vi "Get All Dispatcher Queues.vi"(0 "receiver host (\"\")":string, 5 "receiver port (0)":u16, 11 "error in":errorcluster) -> (4 "response message":T1, 6 "string response":string, 8 "queue names":string[](array[string]), 15 "error out":errorcluster)   [LabVIEW 2013, in "AMC.lvlib"]
doc: "Requests a list of all the queue names in the application instance specified by \"receiver host\" and \"receiver port\".\n\nIf \"receiver port\" is undefined, this VI will attempt to use the default UDP port."
uses:
  AMC.lvlib
  Message.ctl
  <vilib>/NI/Tools/Keyed Array/KeyedArray.ctl
  <vilib>/NI/Tools/Keyed Array/Map String.vi
  <vilib>/NI/Tools/String/Get Case Matching.vi
  Globals.vi
  <vilib>/NI/Tools/Keyed Array/Tools_KeyedArray.lvlib
panel:
  in  "timeout (100 ms)":i32=100
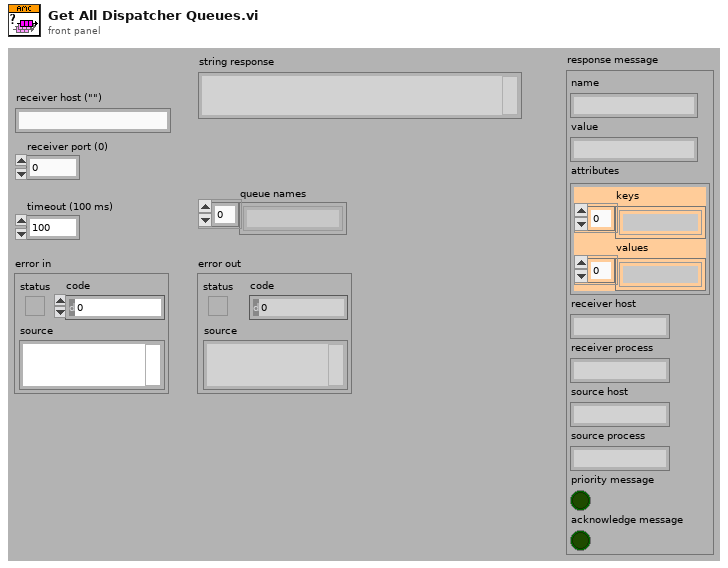
[diagram p1: front panel]
types:
  T1 = typedef "AMC.lvlib/Message.ctl" = cluster{"name":string, "value":string, "attributes":T2, "receiver host":string, "receiver process":string, "source host":string, "source process":string, "priority message":bool, "acknowledge message":bool}
  T2 = typedef "Tools_KeyedArray.lvlib/KeyedArray.ctl" = cluster{"keys":string[], "values":string[]}
  T3 = typedef "AMC.lvlib/Message Queue.ctl" = refnum<queue>
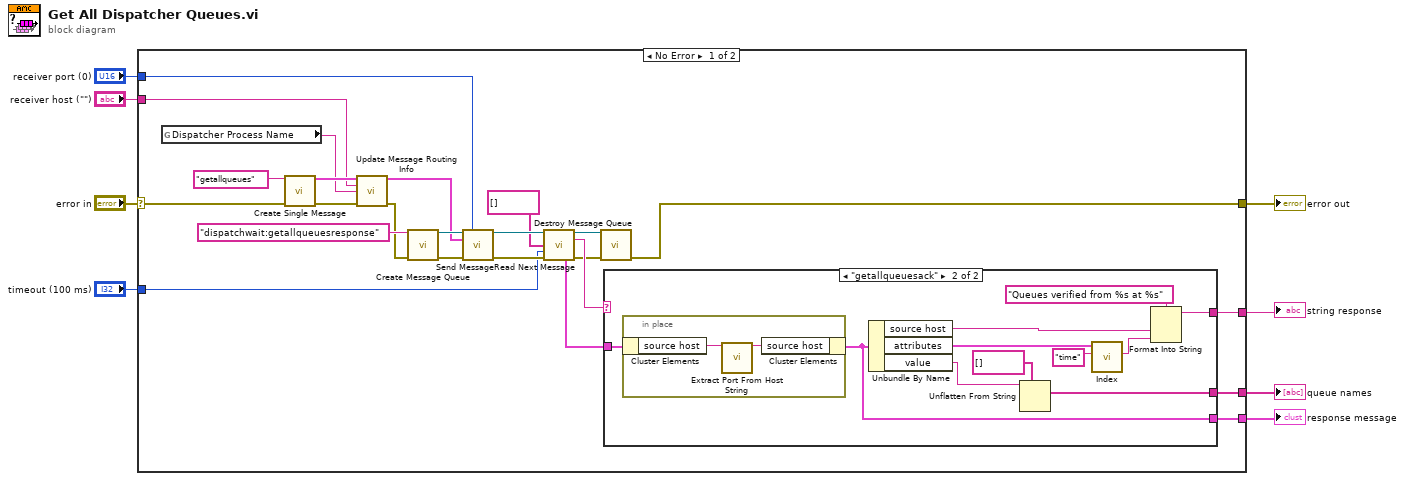
[diagram p0: block diagram]
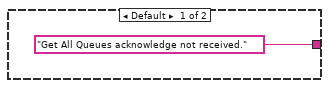
[diagram p2: hidden frame]
diagram:
  n1 = case shown="No Error" "error in" {
    selector: "error in" -> [w12 w47]
    tunnel: [w32 _] -> w8
    tunnel: [w31 w47] -> w7
    tunnel: [w28 _] -> w6
    tunnel: "receiver host (\"\")" -> [w17 _]
    tunnel: "timeout (100 ms)" -> [w9 _]
    tunnel: [w21 _] -> w2
    tunnel: "receiver port (0)" -> [w11 _]
    frame No Error {
      n2 = global read "Globals.vi" "Dispatcher Process Name"() -> (w18:string)
      n3 = call "Create Single Message.vi"("name"="getallqueues" ("Name"), "error in"=w12) -> ("message"=w20:T1, "error out"=w14:errorcluster)  [unwired: 12 in]
      n4 = call "Update Message Routing Info.vi"("message"=w20, "receiver host (\"\")"=w17, "receiver process (\"\")"=w18, "error in"=w14) -> ("message"=w19:T1, "error out"=w13:errorcluster)  [unwired: 10 in]
      n5 = call "Create Message Queue.vi"("message queue name"="dispatchwait:getallqueuesresponse", "error in"=w13) -> ("message queue out"=w25:T3, "error out"=w29:errorcluster)  [unwired: 12 in]
      n6 = call "Send Message.vi"("message queue in"=w25, "receiver port"=w11, "message"=w19, "error in"=w29) -> ("message queue out"=w24:T3, "error out"=w30:errorcluster)  [unwired: 9 in, 1 out]
      n7 = call "Read Next Message.vi"("message queue in"=w24, "termination list ([Exit])"=string[] [], "timeout (1 ms)"=w9, "error in"=w30) -> ("message queue out"=w15:T3, "message name"=w23:string, "message"=w22:T1, "error out"=w16:errorcluster)  [unwired: 4 in, 4 out]
      n8 = call "Destroy Message Queue.vi"("message queue in"=w15, "error in"=w16) -> ("error out"=w31:errorcluster)  [unwired: 11 in, 2 out]
      n9 = case shown="\"getallqueuesack\"" w23 {
        tunnel: w22 -> [_ w35]
        tunnel: ["Get All Queues acknowledge not received." w44] -> w32
        tunnel: [_ w34] -> w28
        tunnel: [_ w36] -> w21
        frame Default {
        }
        frame "getallqueuesack" {
          n10 = in-place {
            n11 = in-place-cluster #1(w35) -> ("source host"=w46:string)
            n12 = call "Extract Port From Host String.vi"("host in"=w46) -> ("host out"=w45:string)  [unwired: 12 in, 2 out]
            n13 = in-place-cluster #1("source host"=w45) -> (w34:T1)
          }
          n14 = Unbundle By Name(w34) -> ("source host"=w40:string, "attributes"=w41:T2, "value"=w38:string)
          n15 = Unflatten From String(type=string[] [], binary string=w38) -> (value=w36:string[])  [unwired: 3 in, 2 out]
          n16 = call <vilib>:"Index.vi"("key"="time", "array in"=w41) -> ("value"=w39:string)  [unwired: 2 in, 3 out]
          n17 = Format Into String(format string="Queues verified from %s at %s", w40, w39) -> (resulting string=w44:string)  [unwired: 2 in, 1 out]
        }
      }
    }
    frame Error {
    }
  }
  "error out" <- w7
  "string response" <- w8
  "response message" <- w6
  "queue names" <- w2
